vi "DPT Panel Reset Gas Volume.vi"(11 "Tasks In":refnum<k21>[](array[refnum])) -> (3 "CDAQ Data Out":dbl[](array[numeric]))   [LabVIEW 2016]
panel:
  in  "ok":bool
  out "message":string="Reset Gas Volume"
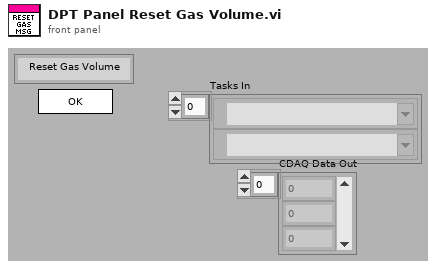
[diagram p1: front panel]
types:
  T1 = enum16{"Exe", "Init CDAQ", "Gather DATA", "Close"}
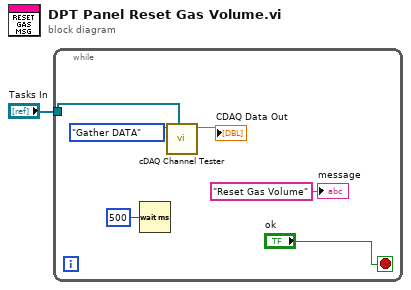
[diagram p0: block diagram]
diagram:
  n1 = while {
    tunnel: "Tasks In" -> [w4]
    stop <- "ok" stop-if-true
    n2 = Wait (ms)(milliseconds to wait=u32 500) -> ()  [unwired: 1 out]
    n3 = call "cDAQ Channel Tester.vi"(7:w4, 11:T1."Gather DATA" ("Mode")) -> (2:→"CDAQ Data Out")  [unwired: 8 in, 1 out]
    "message" <- "Reset Gas Volume" ("message")
  }
